vi "Extract FFT of Real Sequence from FFT Output_Host.vi"() -> ()   [LabVIEW 2011]
uses:
  <userlib>/FPGA Library/Code Development/Signal Processing/FFT/Real Sequence from Complex FFT/BRAM State.ctl
  <instrlib>/FlexRIO/Libraries/Helper VIs/NI FlexRIO Helper VIs.lvlib
panel:
  out "Array 3":u16[](array[numeric])
  out "Output 2":dbl[](array[numeric]) format="%.2f"
  out "Array 2":T1[](array[typedef])
  out "Address":u16[](array[numeric])
  out "Numeric":i32
  out "Output":dbl[](array[numeric]) format="%.2f"
  out "Array":u16[](array[numeric])
  in  "stop":bool
  in  "Input Valid":i16
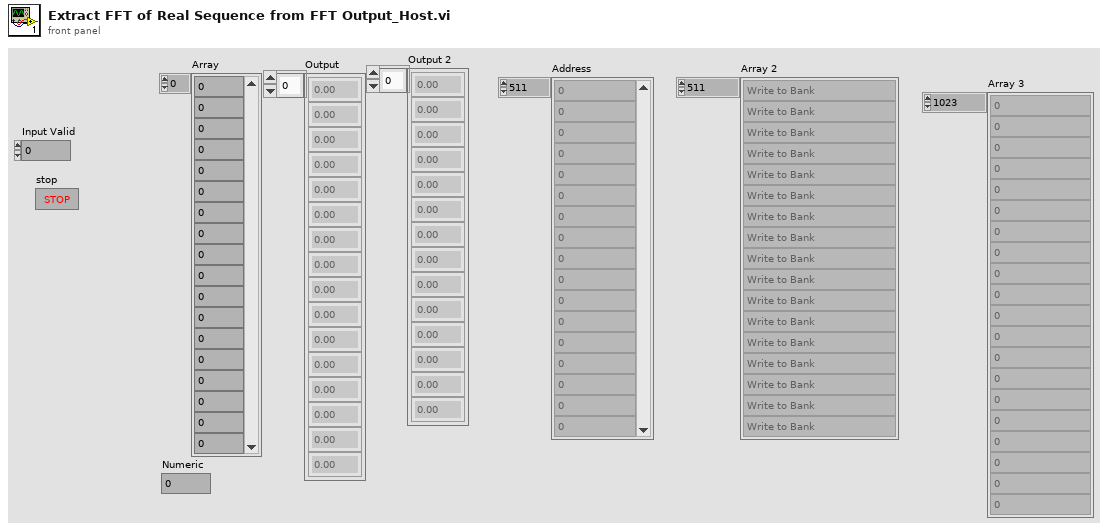
[diagram p1: front panel]
types:
  T1 = typedef "BRAM State.ctl" = enum8{"Write to Bank", "Read from Bank"}
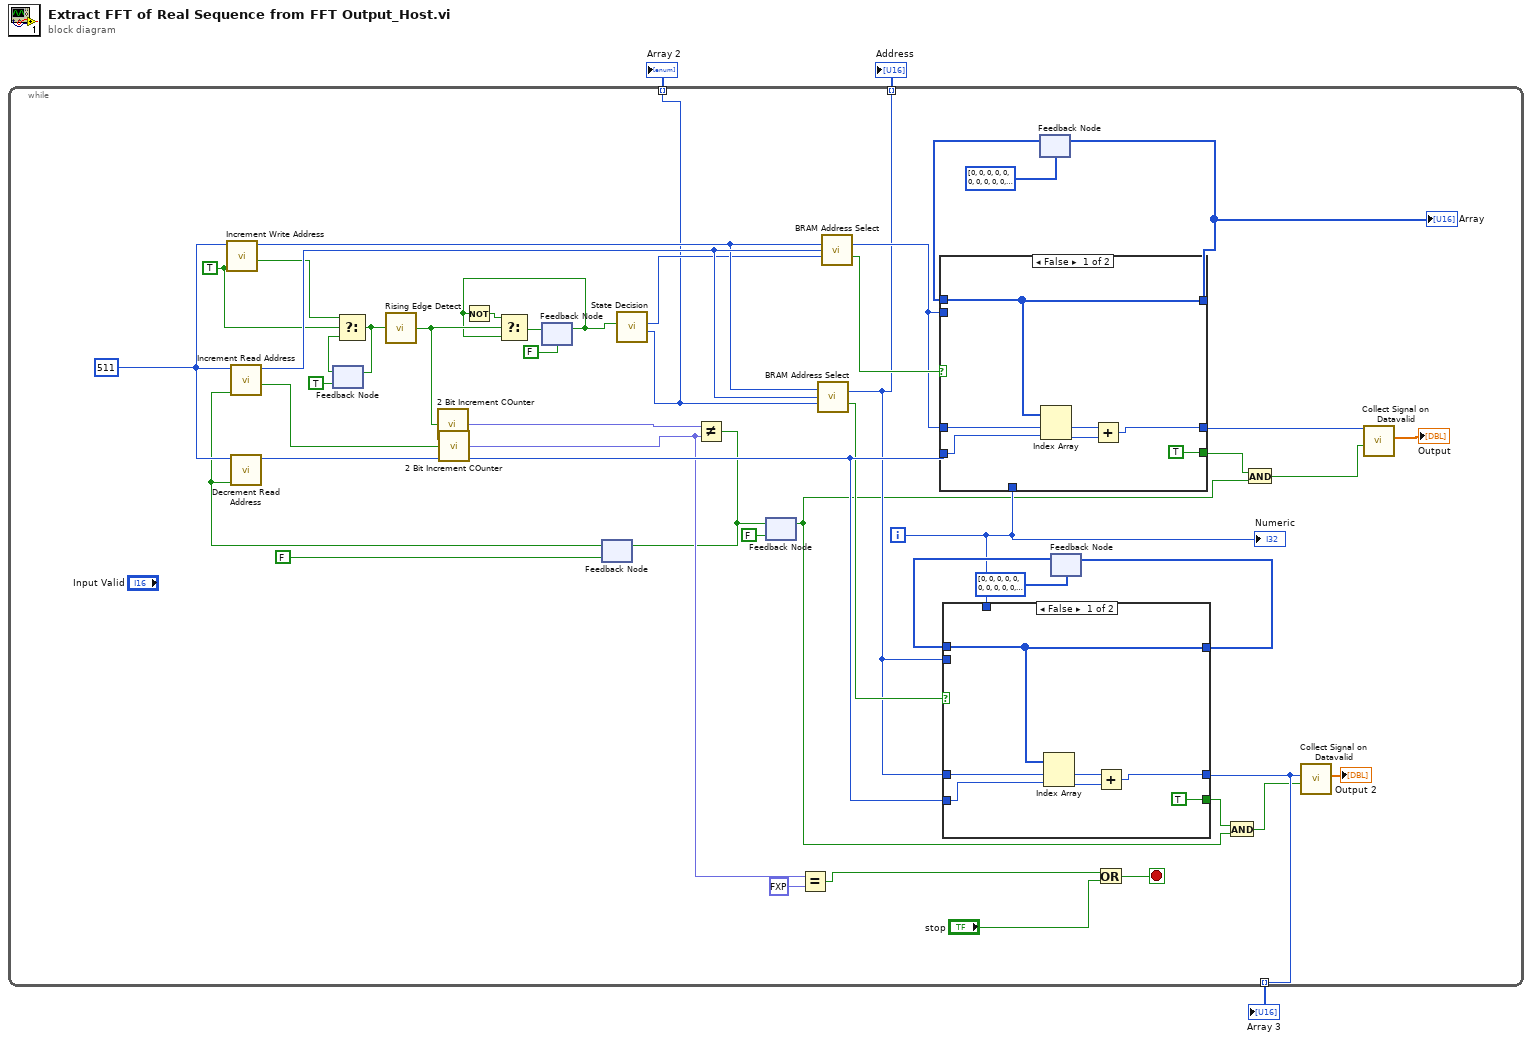
[diagram p0: block diagram]
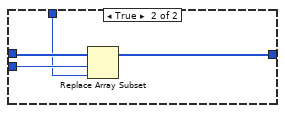
[diagram p2: hidden frame]
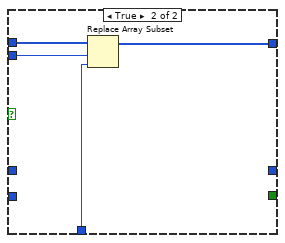
[diagram p3: hidden frame]
diagram:
  n1 = while {
    tunnel: [w15] -> w3 mode=indexing
    tunnel: [w14] -> w2 mode=indexing
    tunnel: [w12] -> w1 mode=indexing
    i -> [w34]
    stop <- w45 stop-if-true
    w25 = TRUE ("INC?")
    w44 = u16 511 ("rollover")
    n2 = call <userlib>:"Increment Write Address.vi"("INC?"=w25, "rollover"=w44) -> ("roll over"=w24:bool, "count"=w28:u16)  [unwired: 8 in]
    n3 = feedback #1(TRUE ("roll over")) -> (w23:bool)
    n4 = Select(t=w24, s=w25, f=w23) -> (s? t:f=w22:bool)
    n5 = feedback-in #1(w22) -> ()
    n6 = call <instrlib>:"Rising Edge Detect.vi"("signal"=w22) -> ("edge detected"=w26:bool)  [unwired: 14 in]
    n7 = call <userlib>:"2 Bit Increment COunter.vi"("Increment"=w26) -> ("Counter Value"=w41:fxp<+,3,3>)  [unwired: 14 in]
    n8 = feedback #2(FALSE) -> (w18:bool)
    n9 = Not(x=w18) -> (.not. x?=w27:bool)
    n10 = Select(t=w27, s=w26, f=w18) -> (s? t:f=w19:bool)
    n11 = feedback-in #2(w19) -> ()
    n12 = feedback #3(FALSE) -> (w7:bool)
    n13 = call <userlib>:"Increment Read Address.vi"("INC?"=w7, "rollover"=w44) -> ("roll over"=w42:bool, "count"=w43:u16)  [unwired: 8 in]
    n14 = call <userlib>:"Decrement Read Address.vi"("DEC?"=w7, "Load Value"=w44) -> ("count"=w37:u16)  [unwired: 8 in, 1 out]
    n15 = call <userlib>:"2 Bit Increment COunter.vi"("Increment"=w42) -> ("Counter Value"=w32:fxp<+,3,3>)  [unwired: 14 in]
    n16 = call <userlib>:"State Decision.vi"("Change?"=w18) -> ("BRAM1 State"=w14:T1, "BRAM0 State"=w16:T1)  [unwired: 9 in]
    n17 = Not Equal?(x=w41, y=w32) -> (x != y?=w6:bool)
    n18 = feedback-in #3(w6) -> ()
    n19 = feedback #4(FALSE) -> (w5:bool)
    n20 = feedback-in #4(w6) -> ()
    n21 = Equal?(x=w32, y=fxp<+,3,3> 2.0) -> (x = y?=w30:bool)
    n22 = call <userlib>:"BRAM Address Select.vi"("Write Address"=w28, "Read Address"=w43, "Read/Write?"=w14) -> ("BRAM Address"=w15:u16, "Write?"=w33:bool)  [unwired: 11 in]
    n23 = call <userlib>:"BRAM Address Select.vi"("Write Address"=w28, "Read Address"=w43, "Read/Write?"=w16) -> ("BRAM Address"=w20:u16, "Write?"=w29:bool)  [unwired: 11 in]
    n24 = feedback #5(u16[] [0, 0, 0, 0, 0, 0, 0, 0, 0, 0, 0, 0, 0, 0, 0, 0, 0, 0, 0, 0, 0, 0, 0, 0, 0, 0, 0, 0, 0, 0, 0, 0, 0, 0, 0, 0, 0, 0, 0, 0, 0, 0, 0, 0, 0, 0, 0, 0, 0, 0, 0, 0, 0, 0, 0, 0, 0, 0, 0, 0, 0, 0, 0, 0, 0, 0, 0, 0, 0, 0, 0, 0, 0, 0, 0, 0, 0, 0, 0, 0, 0, 0, 0, 0, 0, 0, 0, 0, 0, 0, 0, 0, 0, 0, 0, 0, 0, 0, 0, 0, 0, 0, 0, 0, 0, 0, 0, 0, 0, 0, 0, 0, 0, 0, 0, 0, 0, 0, 0, 0, 0, 0, 0, 0, 0, 0, 0, 0, 0, 0, 0, 0, 0, 0, 0, 0, 0, 0, 0, 0, 0, 0, 0, 0, 0, 0, 0, 0, 0, 0, 0, 0, 0, 0, 0, 0, 0, 0, 0, 0, 0, 0, 0, 0, 0, 0, 0, 0, 0, 0, 0, 0, 0, 0, 0, 0, 0, 0, 0, 0, 0, 0, 0, 0, 0, 0, 0, 0, 0, 0, 0, 0, 0, 0, 0, 0, 0, 0, 0, 0, 0, 0, 0, 0, 0, 0, 0, 0, 0, 0, 0, 0, 0, 0, 0, 0, 0, 0, 0, 0, 0, 0, 0, 0, 0, 0, 0, 0, 0, 0, 0, 0, 0, 0, 0, 0, 0, 0, 0, 0, 0, 0, 0, 0, 0, 0, 0, 0, 0, 0, 0, 0, 0, 0, 0, 0, 0, 0, 0, 0, 0, 0, 0, 0, 0, 0, 0, 0, 0, 0, 0, 0, 0, 0, 0, 0, 0, 0, 0, 0, 0, 0, 0, 0, 0, 0, 0, 0, 0, 0, 0, 0, 0, 0, 0, 0, 0, 0, 0, 0, 0, 0, 0, 0, 0, 0, 0, 0, 0, 0, 0, 0, 0, 0, 0, 0, 0, 0, 0, 0, 0, 0, 0, 0, 0, 0, 0, 0, 0, 0, 0, 0, 0, 0, 0, 0, 0, 0, 0, 0, 0, 0, 0, 0, 0, 0, 0, 0, 0, 0, 0, 0, 0, 0, 0, 0, 0, 0, 0, 0, 0, 0, 0, 0, 0, 0, 0, 0, 0, 0, 0, 0, 0, 0, 0, 0, 0, 0, 0, 0, 0, 0, 0, 0, 0, 0, 0, 0, 0, 0, 0, 0, 0, 0, 0, 0, 0, 0, 0, 0, 0, 0, 0, 0, 0, 0, 0, 0, 0, 0, 0, 0, 0, 0, 0, 0, 0, 0, 0, 0, 0, 0, 0, 0, 0, 0, 0, 0, 0, 0, 0, 0, 0, 0, 0, 0, 0, 0, 0, 0, 0, 0, 0, 0, 0, 0, 0, 0, 0, 0, 0, 0, 0, 0, 0, 0, 0, 0, 0, 0, 0, 0, 0, 0, 0, 0, 0, 0, 0, 0, 0, 0, 0, 0, 0, 0, 0, 0, 0, 0, 0, 0, 0, 0, 0, 0, 0, 0, 0, 0, 0, 0, 0, 0, 0, 0, 0, 0, 0, 0, 0, 0, 0, 0, 0, 0, 0, 0, 0, 0, 0, 0] ("initialized array")) -> (w50:u16[])
    n25 = case shown="False" w29 {
      tunnel: [w68 w72] -> w49
      tunnel: w50 -> [w68 w71]
      tunnel: [w64 _] -> w48
      tunnel: [TRUE _] -> w9
      tunnel: w37 -> [w63 _]
      tunnel: w20 -> [w62 _]
      tunnel: w20 -> [_ w70]
      tunnel: w34 -> [_ w69]
      frame False {
        n26 = Index Array(array=w68, index #1=w62, index #2=w63) -> (element #1=w66:u16, element #2=w65:u16)
        n27 = Add(x=w66, y=w65) -> (x+y=w64:u16)
      }
      frame True {
        n28 = Replace Array Subset(array=w71, new element=w69, index=w70) -> (w72:u16[])
      }
    }
    "Array" <- w49
    n29 = feedback-in #5(w49) -> ()
    n30 = feedback #6(u16[] [0, 0, 0, 0, 0, 0, 0, 0, 0, 0, 0, 0, 0, 0, 0, 0, 0, 0, 0, 0, 0, 0, 0, 0, 0, 0, 0, 0, 0, 0, 0, 0, 0, 0, 0, 0, 0, 0, 0, 0, 0, 0, 0, 0, 0, 0, 0, 0, 0, 0, 0, 0, 0, 0, 0, 0, 0, 0, 0, 0, 0, 0, 0, 0, 0, 0, 0, 0, 0, 0, 0, 0, 0, 0, 0, 0, 0, 0, 0, 0, 0, 0, 0, 0, 0, 0, 0, 0, 0, 0, 0, 0, 0, 0, 0, 0, 0, 0, 0, 0, 0, 0, 0, 0, 0, 0, 0, 0, 0, 0, 0, 0, 0, 0, 0, 0, 0, 0, 0, 0, 0, 0, 0, 0, 0, 0, 0, 0, 0, 0, 0, 0, 0, 0, 0, 0, 0, 0, 0, 0, 0, 0, 0, 0, 0, 0, 0, 0, 0, 0, 0, 0, 0, 0, 0, 0, 0, 0, 0, 0, 0, 0, 0, 0, 0, 0, 0, 0, 0, 0, 0, 0, 0, 0, 0, 0, 0, 0, 0, 0, 0, 0, 0, 0, 0, 0, 0, 0, 0, 0, 0, 0, 0, 0, 0, 0, 0, 0, 0, 0, 0, 0, 0, 0, 0, 0, 0, 0, 0, 0, 0, 0, 0, 0, 0, 0, 0, 0, 0, 0, 0, 0, 0, 0, 0, 0, 0, 0, 0, 0, 0, 0, 0, 0, 0, 0, 0, 0, 0, 0, 0, 0, 0, 0, 0, 0, 0, 0, 0, 0, 0, 0, 0, 0, 0, 0, 0, 0, 0, 0, 0, 0, 0, 0, 0, 0, 0, 0, 0, 0, 0, 0, 0, 0, 0, 0, 0, 0, 0, 0, 0, 0, 0, 0, 0, 0, 0, 0, 0, 0, 0, 0, 0, 0, 0, 0, 0, 0, 0, 0, 0, 0, 0, 0, 0, 0, 0, 0, 0, 0, 0, 0, 0, 0, 0, 0, 0, 0, 0, 0, 0, 0, 0, 0, 0, 0, 0, 0, 0, 0, 0, 0, 0, 0, 0, 0, 0, 0, 0, 0, 0, 0, 0, 0, 0, 0, 0, 0, 0, 0, 0, 0, 0, 0, 0, 0, 0, 0, 0, 0, 0, 0, 0, 0, 0, 0, 0, 0, 0, 0, 0, 0, 0, 0, 0, 0, 0, 0, 0, 0, 0, 0, 0, 0, 0, 0, 0, 0, 0, 0, 0, 0, 0, 0, 0, 0, 0, 0, 0, 0, 0, 0, 0, 0, 0, 0, 0, 0, 0, 0, 0, 0, 0, 0, 0, 0, 0, 0, 0, 0, 0, 0, 0, 0, 0, 0, 0, 0, 0, 0, 0, 0, 0, 0, 0, 0, 0, 0, 0, 0, 0, 0, 0, 0, 0, 0, 0, 0, 0, 0, 0, 0, 0, 0, 0, 0, 0, 0, 0, 0, 0, 0, 0, 0, 0, 0, 0, 0, 0, 0, 0, 0, 0, 0, 0, 0, 0, 0, 0, 0, 0, 0, 0, 0, 0, 0, 0, 0, 0, 0, 0, 0, 0, 0, 0, 0, 0, 0, 0, 0, 0, 0, 0, 0, 0, 0, 0, 0, 0, 0, 0, 0] ("initialized array")) -> (w39:u16[])
    n31 = case shown="False" w33 {
      tunnel: [w57 w61] -> w38
      tunnel: w39 -> [w57 w60]
      tunnel: [w55 _] -> w12
      tunnel: [TRUE _] -> w11
      tunnel: w37 -> [w54 _]
      tunnel: w15 -> [w53 _]
      tunnel: w15 -> [_ w59]
      tunnel: w34 -> [_ w58]
      frame False {
        n32 = Index Array(array=w57, index #1=w53, index #2=w54) -> (element #1=w52:u16, element #2=w51:u16)
        n33 = Add(x=w52, y=w51) -> (x+y=w55:u16)
      }
      frame True {
        n34 = Replace Array Subset(array=w60, new element=w58, index=w59) -> (w61:u16[])
      }
    }
    n35 = feedback-in #6(w38) -> ()
    n36 = Or(x=w30, y="stop") -> (x .or. y?=w45:bool)
    n37 = And(x=w11, y=w5) -> (x .and. y?=w10:bool)
    n38 = And(x=w9, y=w5) -> (x .and. y?=w8:bool)
    n39 = call <userlib>:"Collect Signal on Datavalid.vi"("Data Valid"=w10, "Input"=w12) -> ("Output"=→"Output 2":dbl[])  [unwired: 9 in]
    n40 = call <userlib>:"Collect Signal on Datavalid.vi"("Data Valid"=w8, "Input"=w48) -> ("Output"=→"Output":dbl[])  [unwired: 9 in]
    "Numeric" <- w34
  }
  "Address" <- w3
  "Array 2" <- w2
  "Array 3" <- w1
